vi "5492_PixelHeightCheck.vi"(5 "Margin of Error":i32, 7 "Pixel Goal":dbl) -> (2 "Highest Height":dbl, 3 "Goal Achieved":bool)   [LabVIEW 2016]
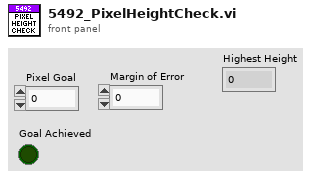
[diagram p1: front panel]
types:
  T1 = cluster{"centerX":dbl[], "centerY":dbl[], "area":dbl[], "width":dbl[], "height":dbl[], "solidity":dbl[]}
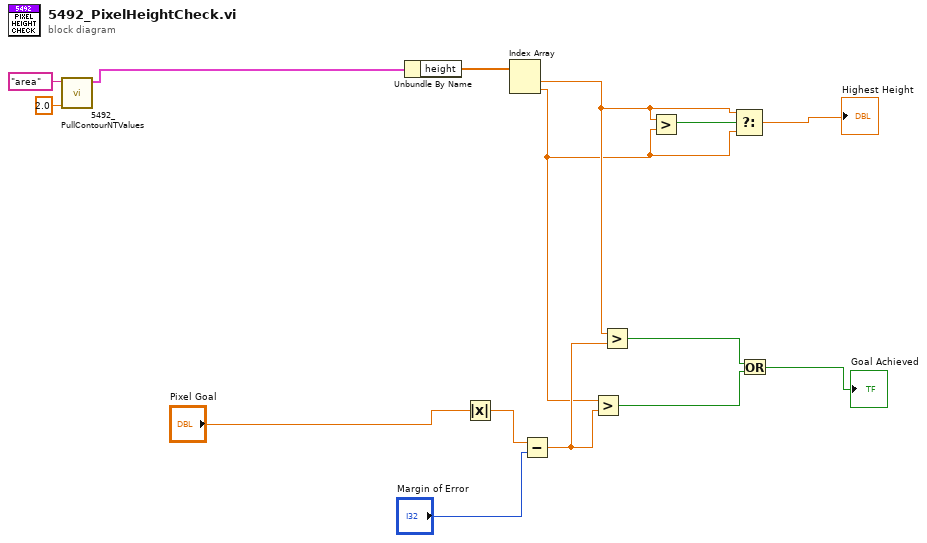
[diagram p0: block diagram]
diagram:
  n1 = call "5492_PullContourNTValues.vi"("Shapes Found"=2.0, "Max Value\nMax Value"="area" ("Max Value\nMax Value")) -> ("Output Cluster"=w10:T1)  [unwired: 9 in]
  n2 = Unbundle By Name(w10) -> ("height"=w9:dbl[])
  n3 = Absolute Value(x="Pixel Goal") -> (abs(x)=w13:dbl)
  n4 = Index Array(array=w9) -> (element #1=w4:dbl, element #2=w3:dbl)  [unwired: 2 in]
  n5 = Subtract(x=w13, y="Margin of Error") -> (x-y=w5:dbl)
  n6 = Greater?(x=w3, y=w5) -> (0:w8:bool)
  n7 = Greater?(x=w4, y=w5) -> (0:w6:bool)
  n8 = Greater?(x=w4, y=w3) -> (0:w1:bool)
  n9 = Select(t=w4, s=w1, f=w3) -> (s? t:f=→"Highest Height":dbl)
  n10 = Or(x=w6, y=w8) -> (x .or. y?=→"Goal Achieved":bool)
